vi "Split Path Segments.vi"(4 "Path String":string) -> (7 "Path Segments":string[](array[string]))   [LabVIEW 2020, in "URI.lvlib"]
uses:
  URI.lvlib
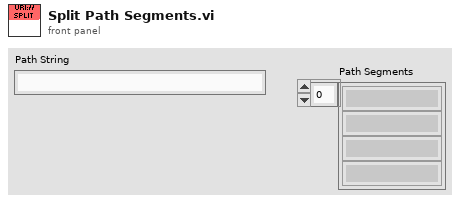
[diagram p1: front panel]
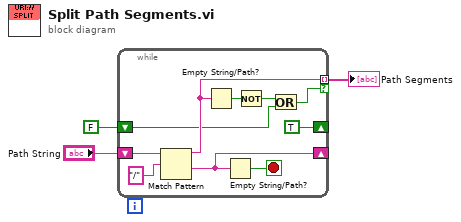
[diagram p0: block diagram]
diagram:
  n1 = while {
    shift-right: [w9] -> _
    shift-left: "Path String" -> [w13]
    tunnel: [w11] -> w2 mode=indexing if=w6
    shift-right: [TRUE] -> _
    shift-left: FALSE -> [w4]
    stop <- w8 stop-if-true
    n2 = Match Pattern(string=w13, regular expression="/") -> (before substring=w11:string, after substring=w9:string)  [unwired: 1 in, 2 out]
    n3 = Empty String/Path?(string/path=w11) -> (empty?=w10:bool)
    n4 = Empty String/Path?(string/path=w9) -> (empty?=w8:bool)
    n5 = Not(x=w10) -> (.not. x?=w7:bool)
    n6 = Or(x=w7, y=w4) -> (x .or. y?=w6:bool)
  }
  "Path Segments" <- w2
